vi "Create.vi"(6 "Labels":map{string, string}(c390), 7 "Registry Name":string="_default_registry", 8 "error in (no error)":errorcluster) -> (0 "error out":errorcluster, 3 "LabVIEW Collector out":refnum<class "LabVIEW Collector.lvclass">)   [LabVIEW 2020, in "Collector.lvlib" / "LabVIEW Collector.lvclass"]
uses:
  LabVIEW Collector.lvclass
  metrics/gauge/Gauge.lvclass
  C:/Github-locals/PromVIEW/src/metrics/metric/Metric.lvclass
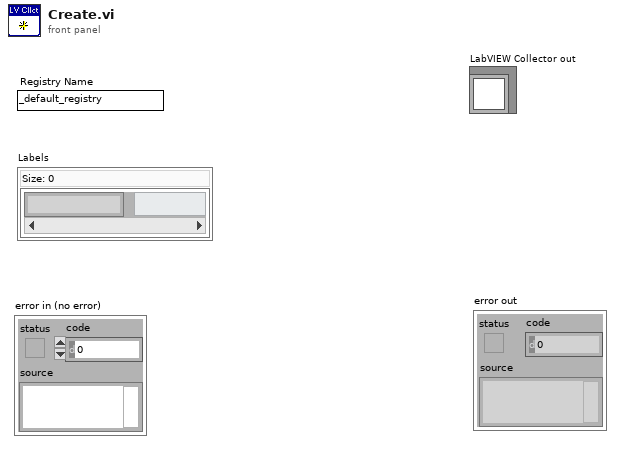
[diagram p1: front panel]
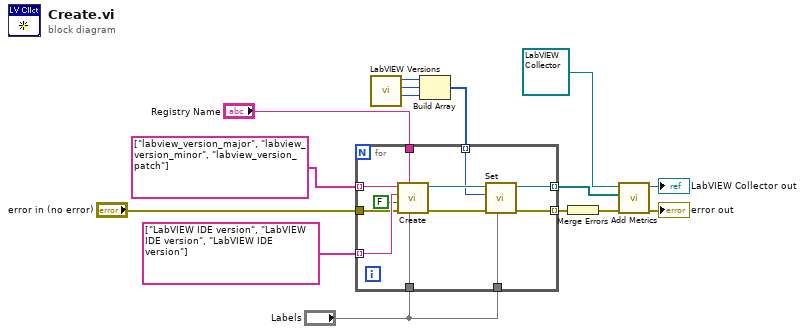
[diagram p0: block diagram]
diagram:
  n1 = call "LabVIEW Versions.vi"() -> ("Patch"=w12:i32, "Minor"=w13:i32, "Major"=w14:i32)  [unwired: 9 in]
  n2 = Build Array(w14, w13, w12) -> (w11:i32[])
  n3 = for {
    tunnel: string[] ["labview_version_major", "labview_version_minor", "labview_version_patch"] ("Metric Name") -> [w26] mode=indexing
    tunnel: w11 -> [w25] mode=indexing
    tunnel: string[] ["LabVIEW IDE version", "LabVIEW IDE version", "LabVIEW IDE version"] ("Metric Name") -> [w24] mode=indexing
    tunnel: "Registry Name" -> [w23]
    tunnel: "Labels" -> [w22]
    tunnel: "Labels" -> [w21]
    tunnel: [w20] -> w7 mode=indexing
    tunnel: [w19] -> w5 mode=indexing
    tunnel: "error in (no error)" -> [w18]
    n4 = call "Create.vi"("Labels"=w22, "Registry Name"=w23, "error in (no error)"=w18, "Auto-register?"=FALSE, "Description"=w24, "Metric Name"=w26) -> ("error out"=w17:errorcluster, "Gauge Ref"=w27:refnum<data-value>)  [unwired: 4 in]
    n5 = call "Set.vi"("Labels"=w21, "error in (no error)"=w17, "Value"=w25, "Gauge Ref"=w27) -> ("error out"=w19:errorcluster, "Gauge Ref out"=w20:refnum<data-value>)  [unwired: 6 in]
  }
  n6 = Merge Errors(w5) -> (w4:errorcluster)
  n7 = call-dynamic "Add Metrics.vi"("error in (no error)"=w4, "Metrics"=w7, "Default Collector in"=refnum<class "LabVIEW Collector.lvclass"> refnum ("Collector.lvlib:LabVIEW Collector.lvclass")) -> ("error out"=→"error out":errorcluster, "Default Collector out"=→"LabVIEW Collector out":refnum<class "LabVIEW Collector.lvclass">)  [unwired: 7 in]
